vi "HandleInput.vi"(8 "error in (no error)":errorcluster, 10 "TeleopInstruction":T1) -> (0 "error out":errorcluster)   [LabVIEW 2013]
uses:
  TeleopInstruction.ctl
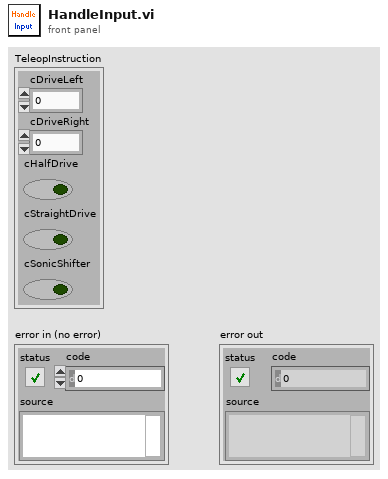
[diagram p1: front panel]
types:
  T1 = typedef "TeleopInstruction.ctl" = cluster{"cDriveLeft":dbl, "cDriveRight":dbl, "cHalfDrive":bool, "cStraightDrive":bool, "cSonicShifter":bool}
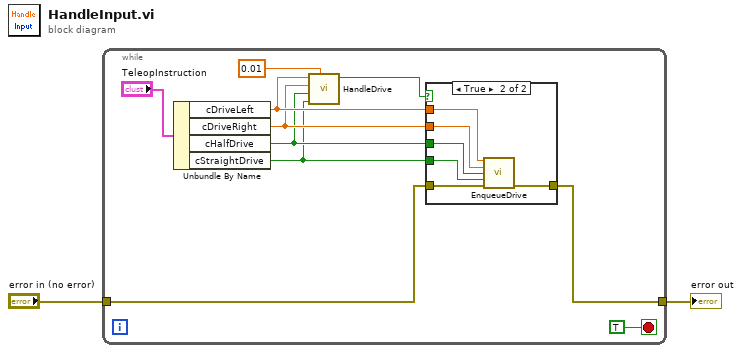
[diagram p0: block diagram]
diagram:
  n1 = while {
    tunnel: "error in (no error)" -> [w5]
    tunnel: [w4] -> w2
    stop <- TRUE stop-if-true
    n2 = Unbundle By Name("TeleopInstruction") -> ("cDriveLeft"=w9:dbl, "cDriveRight"=w8:dbl, "cHalfDrive"=w7:bool, "cStraightDrive"=w6:bool)
    n3 = call "HandleDrive.vi"("Sensitivity"=0.01, "StraightDrive"=w6, "HalfDrive"=w7, "RightMotor"=w8, "LeftMotor"=w9) -> ("Enqueue?"=w3:bool)  [unwired: 6 in]
    n4 = case shown="True" w3 {
      tunnel: w9 -> [_ w19]
      tunnel: w8 -> [_ w18]
      tunnel: w7 -> [_ w17]
      tunnel: w6 -> [_ w16]
      tunnel: w5 -> [w13 w15]
      tunnel: [w13 w14] -> w4
      frame False {
      }
      frame True {
        n5 = call "EnqueueDrive.vi"("cDriveLeft"=w19, "cDriveRight"=w18, "cHalfDrive"=w17, "cStraightDrive"=w16, "error in (no error)"=w15) -> ("error out"=w14:errorcluster)  [unwired: 10 in]
      }
    }
  }
  "error out" <- w2
